vi "Definition Cluster.vi"(11 "Integer in":refnum<class "Integer.lvclass">) -> (2 "Definition":variant, 3 "Integer out":refnum<class "Integer.lvclass">)   [LabVIEW 2020, in "Conditu2.lvlib" / "Columns.lvlib" / "Integer.lvclass"]
uses:
  Integer.lvclass
  C:/dev/lv20CE/lv-conditum-tools/Conditum-Clone/Columns/Type/Type.lvclass
  Integer Definition.ctl
  Type/Definition.ctl
  Attributes.ctl
  Definition.ctl
  Integer.lvclass/Integer.ctl
  Conditu2.lvlib
  Type/Type.lvclass
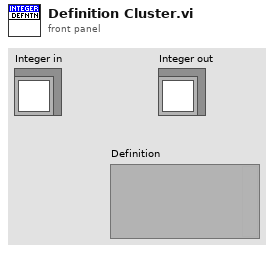
[diagram p1: front panel]
types:
  T1 = typedef "Conditu2.lvlib/Columns.lvlib/Integer.lvclass/Integer Definition.ctl" = cluster{"Type":T2, "Attributes":T3, "Integer":T4}
  T2 = typedef "Conditu2.lvlib/Columns.lvlib/Type.lvclass/Definition.ctl" = cluster{"Name":string, "Nullable":bool, "Default NULL":bool}
  T3 = typedef "Conditu2.lvlib/Attributes.ctl" = cluster{"Primary Key":bool, "Unique":bool, "Foreign Key":bool, "Auto Increment":bool}
  T4 = typedef "Conditu2.lvlib/Columns.lvlib/Integer.lvclass/Definition.ctl" = cluster{"Default":i64}
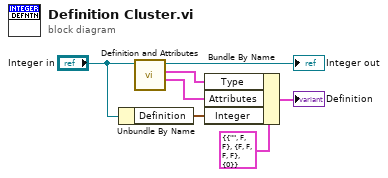
[diagram p0: block diagram]
diagram:
  n1 = Unbundle By Name("Integer in") -> ("Definition"=w6:T4)
  n2 = call "Definition and Attributes.vi"("Type in"="Integer in") -> ("Attributes"=w4:T3, "Definition"=w5:T2, "Type out"=→"Integer out":refnum<class "Integer.lvclass">)  [unwired: 8 in]
  n3 = Bundle By Name(cluster=T1 {"Type"={"Name"="", "Nullable"=FALSE, "Default NULL"=FALSE}, "Attributes"={"Primary Key"=FALSE, "Unique"=FALSE, "Foreign Key"=FALSE, "Auto Increment"=FALSE}, "Integer"={"Default"=0}} ("Integer Definition"), "Type"=w5, "Attributes"=w4, "Integer"=w6) -> (→"Definition":T1)
